vi "Generate hybrid DNA FEC.vi"(0 "dF (pN)":dbl=0.2, 2 "End Force (pN)":dbl, 3 "ssDNA Length (nt)":dbl, 5 "dsDNA Length (bp)":dbl) -> (1 "expected contour length for dsDNA (nm)":dbl, 4 "expected contour length for ssDNA (nm) 2":dbl, 6 "Extension array (nm)":dbl[](array[numeric]), 8 "Force Array (pN)":dbl[](array[numeric]))   [LabVIEW 2014]
panel:
  in  "Tab Control":enum32{"Page 3", "Page 1"}(tab)
  out "XY Graph 2":cluster{dbl[], dbl[]}(graph)
  in  "Start Force (pN)":dbl=0.05
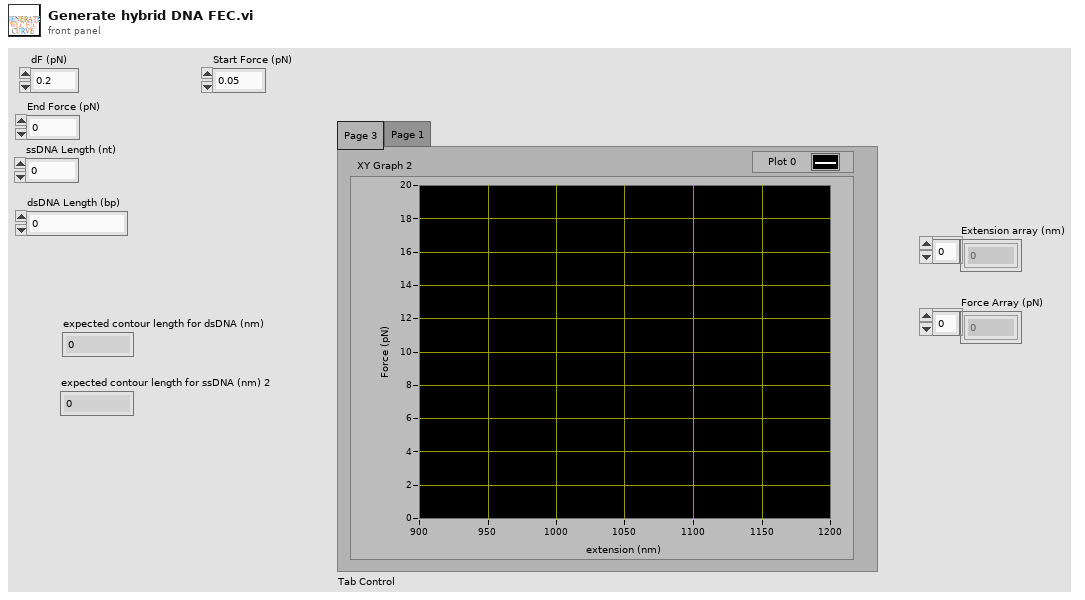
[diagram p1: front panel]
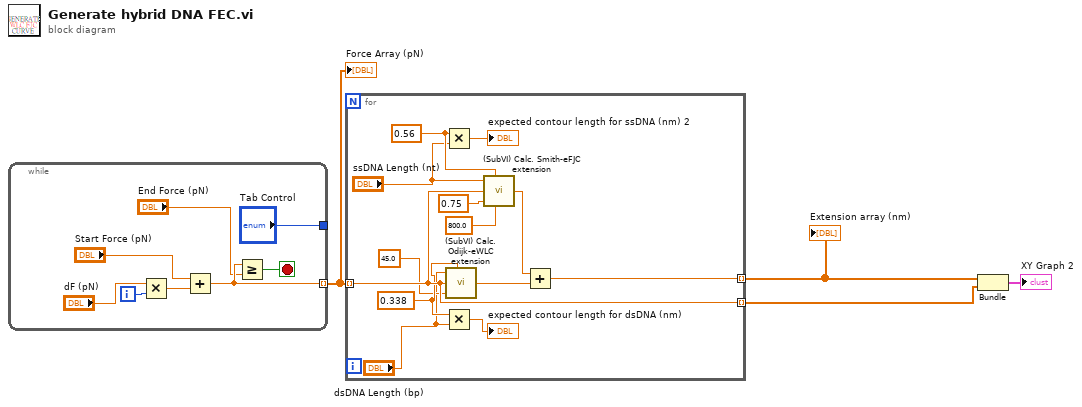
[diagram p0: block diagram]
diagram:
  n1 = while {
    tunnel: [w8] -> w4 mode=indexing
    tunnel: ["Tab Control"] -> _
    i -> [w11]
    stop <- w6 stop-if-true
    n2 = Multiply(x="dF (pN)", y=w11) -> (x*y=w10:dbl)
    n3 = Add(x="Start Force (pN)", y=w10) -> (x+y=w8:dbl)
    n4 = Greater Or Equal?(x=w8, y="End Force (pN)") -> (x >= y?=w6:bool)
  }
  "Force Array (pN)" <- w4
  n5 = for {
    tunnel: w4 -> [w22] mode=indexing
    tunnel: [w23] -> w2 mode=indexing
    tunnel: [w22] -> w3 mode=indexing
    w19 = 0.338 ("nm/bp")
    w17 = 0.56 ("nm/nt")
    n6 = Multiply(x=w17, y="ssDNA Length (nt)") -> (x*y=→"expected contour length for ssDNA (nm) 2":dbl)
    n7 = Multiply(x=w19, y="dsDNA Length (bp)") -> (x*y=→"expected contour length for dsDNA (nm)":dbl)
    n8 = call "(SubVI) Calc. Odijk-eWLC extension.vi"("dsDNA Length (bp)"="dsDNA Length (bp)", "nm/bp"=w19, "Force (pN)"=w22, "Persistence length (nm)"=45.0) -> ("Extension (nm)"=w24:dbl)  [unwired: 3 in]
    n9 = call "(SubVI) Calc. Smith-eFJC extension.vi"("ssDNA Length (nt)"="ssDNA Length (nt)", "nm/nt"=w17, "Force (pN)"=w22, "Persistence length (nm)"=0.75, "Elastic modulus (pN)"=800.0) -> ("Extension (nm)"=w25:dbl)  [unwired: 2 in]
    n10 = Add(x=w25, y=w24) -> (x+y=w23:dbl)
  }
  "Extension array (nm)" <- w2
  n11 = Bundle(w2, w3) -> (→"XY Graph 2":cluster{dbl[], dbl[]})  [unwired: 1 in]
